vi "Read Autostop Nested Actor Count.vi"(11 "Actor in":refnum<class "Actor.lvclass">) -> (2 "Count":i32)   [LabVIEW 2020, in "Actor Framework.lvlib" / "Actor.lvclass"]
doc: "<p>(<strong>Filename</strong>: <span class=\"dnl\">Actor Framework.lvlib:Actor.lvclass:Read Autostop Nested Actor Count.vi</span>)</p>\n\n<p>Returns the number of auto-stop nested actors that were launched by an actor but have not yet sent back their Last Ack messages. Use this VI to detect whether all nested actors have finished working.</p>"
uses:
  Actor.lvclass
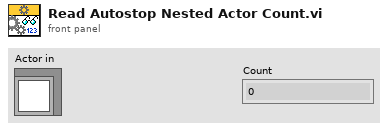
[diagram p1: front panel]
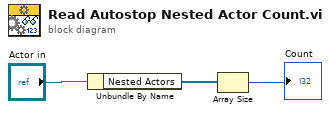
[diagram p0: block diagram]
diagram:
  n1 = Unbundle By Name("Actor in") -> ("Nested Actors"=w2:refnum<class "Message Enqueuer.lvclass">[])
  n2 = Array Size(array=w2) -> (size(s)=→"Count":i32)
